vi "Argument_Exists.vi"(1 "Argument":string, 2 "Argument List":string[](array[string])) -> (0 "Argument Exists":bool)   [LabVIEW 2011]
doc: "This VI is a simple macro that examines the supplied argument list (a string array) and tries to locate a match corresponding to the contents of the \"Argument\" parameter. If a match is found, \"Argument Exists\" returns true."
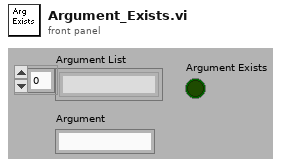
[diagram p1: front panel]
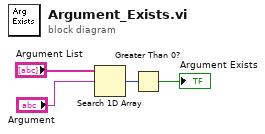
[diagram p0: block diagram]
diagram:
  n1 = Search 1D Array(1D array="Argument List", element="Argument") -> (index of element=w2:i32)  [unwired: 1 out]
  n2 = Greater Than 0?(x=w2) -> (x > 0?=→"Argument Exists":bool)
